vi "2016-120_Measure Device Voltages.vi"(8 "error in (no error)":errorcluster, 11 "DMM_COMPort":i32) -> (0 "error out":errorcluster, 3 "Measurement Data":dbl[](array[numeric]))   [LabVIEW 2015]
doc: "This VI measure power supplies from the Modis Charger Main Board with Keithley DMM."
uses:
  <instrlib>/Keithley 27XX/Public/Data/Read Multiple Direct.vi
  <instrlib>/Keithley 27XX/Keithley 27XX.lvlib
panel:
  in  "Serial Configuration":T1={"Baud Rate (19200)"=19200, "Flow Control (1: XON/XOFF)"=1, "Termination Char (0:CR)"=0} {"Termination Char (0:CR)" items=["CR", "LF"]; "Flow Control (1: XON/XOFF)" items=["None", "XON/XOFF", "RTS/CTS (2701 Only)", "XON/XOFF & RTS/CTS (2701 Only)"]; "Baud Rate (19200)" items=["300"=300, "600"=600, "1200"=1200, "2400"=2400, "4800"=4800, "9600"=9600, "19.2k"=19200, "38.4k (2701 Only)"=38400, "57.6k (2701 Only)"=57600, "115.2k (2701 Only)"=115200]}
  in  "Timeout (5000 milliseconds)":u32=10000
  in  "Function (0: DC Voltage)":u16(ring) items=["DC Voltage", "AC Voltage", "DC Current", "AC Current", "Resistance", "Four-Wire Resistance", "Temperature (C)", "Frequency", "Period", "Continuity"]
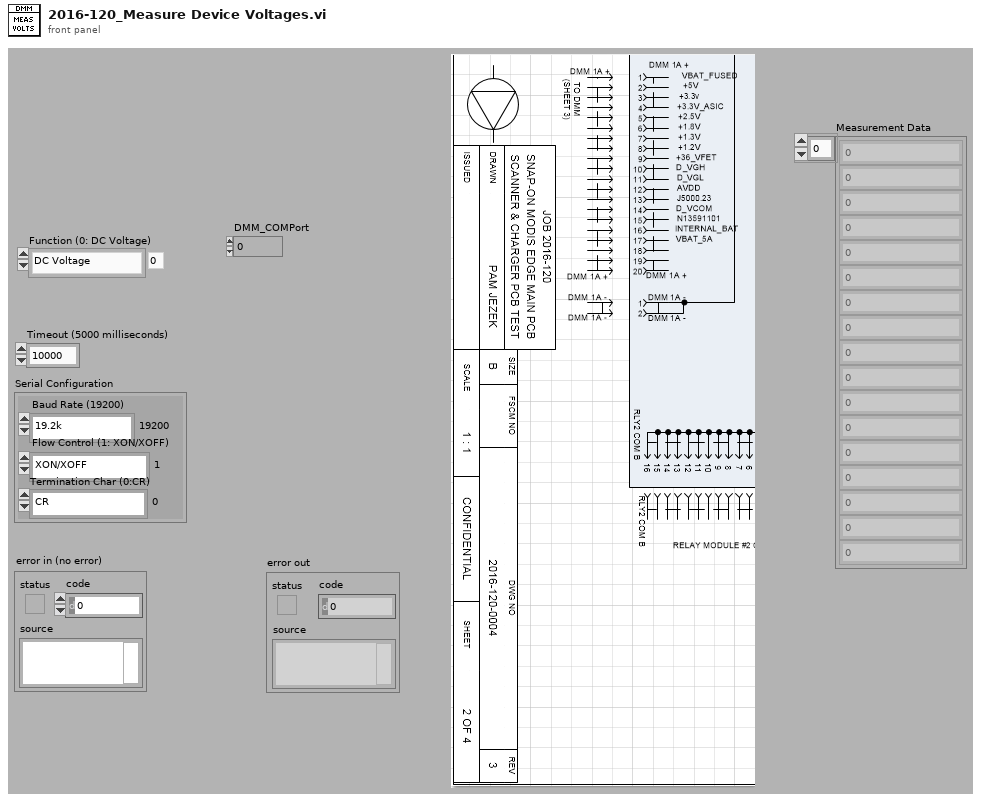
[diagram p1: front panel]
types:
  T1 = cluster{"Baud Rate (19200)":u32, "Flow Control (1: XON/XOFF)":u16, "Termination Char (0:CR)":u16}
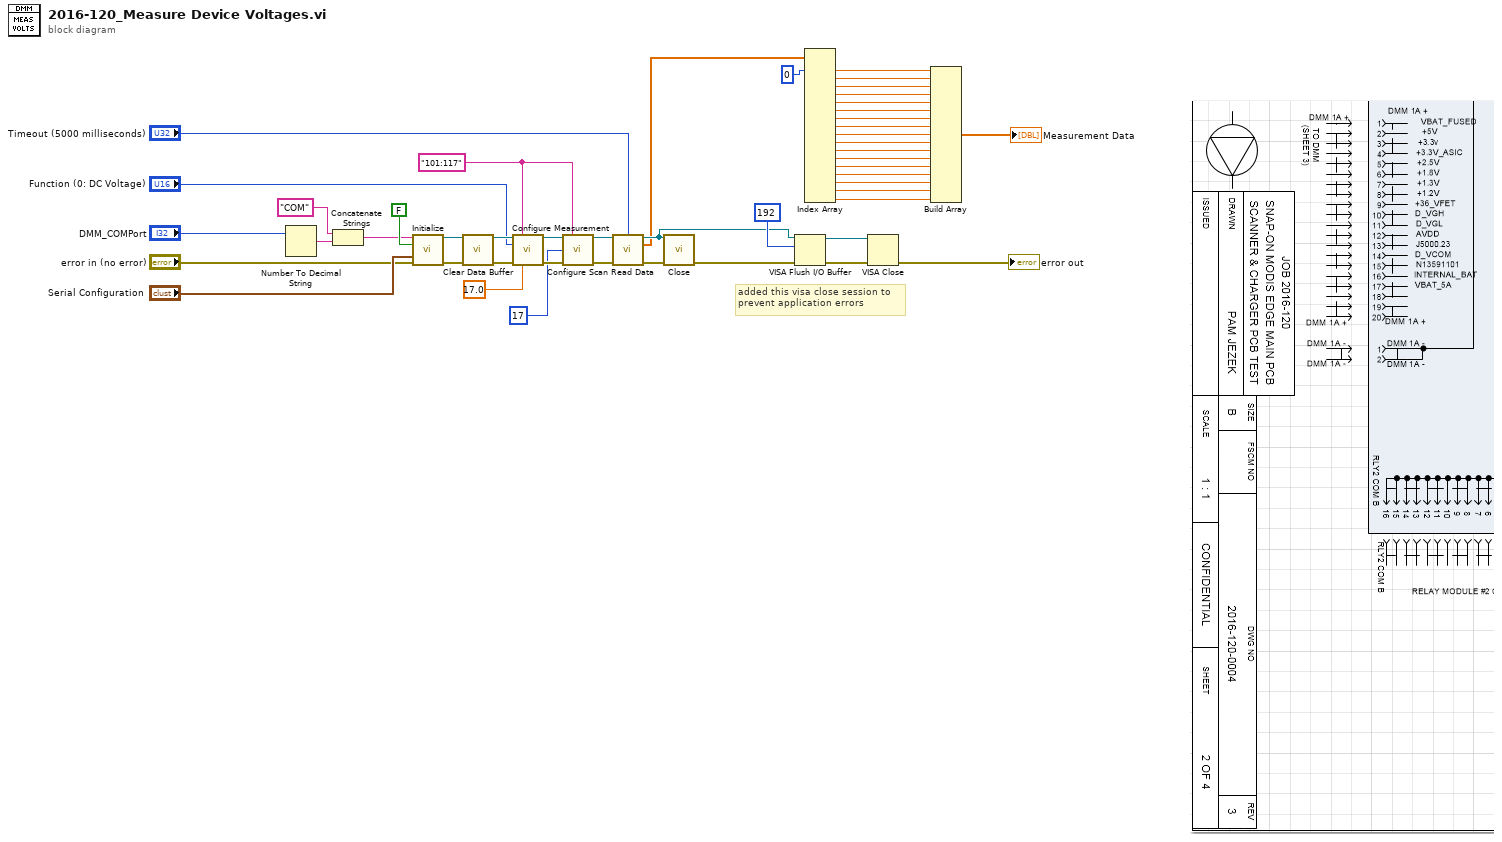
[diagram p0: block diagram]
diagram:
  w36 = "101:117" ("Channel List (101:110)")
  # "added this visa close session to \nprevent application errors"
  n1 = Number To Decimal String(number="DMM_COMPort") -> (decimal integer string=w29:string)  [unwired: 1 in]
  n2 = Concatenate Strings("COM" ("string"), w29) -> (w28:string)
  n3 = call <instrlib>:"Initialize.vi"("VISA resource name"=w28, "ID Query? (T: Yes)"=FALSE, "Serial Configuration"="Serial Configuration", "error in (no error)"="error in (no error)") -> ("VISA resource name out"=w42:refnum<visa-resource-name>, "error out"=w43:errorcluster)  [unwired: 10 in]
  n4 = call <instrlib>:"Clear Data Buffer.vi"("VISA resource name"=w42, "error in (no error)"=w43) -> ("VISA resource name out"=w45:refnum<visa-resource-name>, "error out"=w44:errorcluster)  [unwired: 12 in]
  n5 = call <instrlib>:"Configure Measurement.vi"("VISA resource name"=w45, "Scan List (Empty)"=w36, "Function (0: DC Voltage)"="Function (0: DC Voltage)", "error in (no error)"=w44, "Manual Range (10)"=17.0) -> ("VISA resource name out"=w47:refnum<visa-resource-name>, "error out"=w46:errorcluster)  [unwired: 9 in]
  n6 = call <instrlib>:"Configure Scan.vi"("VISA resource name"=w47, "Channel List (101:110)"=w36, "Sample Count (100)"=17 ("Sample Count (1)"), "error in (no error)"=w46) -> ("VISA resource name out"=w40:refnum<visa-resource-name>, "error out"=w41:errorcluster)  [unwired: 10 in]
  n7 = call-poly <instrlib>:"Read Data.vi"("VISA resource name"=w40, "Timeout (30000 milliseconds)"="Timeout (5000 milliseconds)", "error in (no error)"=w41) -> ("VISA resource name out"=w21:refnum<visa-resource-name>, "Measurement Data"=w2:dbl[], "error out"=w32:errorcluster)  [unwired: 7 in, 3 out]
  n8 = call <instrlib>:"Close.vi"("VISA resource name"=w21, "error in (no error)"=w32) -> ("error out"=w23:errorcluster)  [unwired: 13 in]
  n9 = VISA Flush I/O Buffer(VISA resource name=w21, mask (16)=u16 192, error in (no error)=w23) -> (VISA resource name out=w24:refnum<visa-resource-name>, error out=w26:errorcluster)
  n10 = Index Array(array=w2, index #1=0 ("index")) -> (element #1=w20:dbl, element #2=w19:dbl, element #3=w18:dbl, element #4=w17:dbl, element #5=w16:dbl, element #6=w15:dbl, element #7=w14:dbl, element #8=w13:dbl, element #9=w12:dbl, element #10=w11:dbl, element #11=w10:dbl, element #12=w9:dbl, element #13=w8:dbl, element #14=w7:dbl, element #15=w5:dbl, element #16=w6:dbl, element #17=w4:dbl)  [unwired: 16 in]
  n11 = VISA Close(VISA resource name=w24, error in (no error)=w26) -> (error out=→"error out":errorcluster)
  n12 = Build Array(w20, w19, w18, w17, w16, w15, w14, w13, w12, w11, w10, w9, w8, w7, w5, w6, w4) -> (→"Measurement Data":dbl[])
